vi "Populate 32-bit Block Memory.vi"(9 "Number of U32 words in Array":i32, 10 "Boolean array Block Mem in":refnum<k21>="Boolean Array", 11 "U32 Block Mem in":refnum<k21>) -> (3 "U32 Block mem Out":refnum<k21>)   [LabVIEW 2014]
uses:
  <vilib>/rvi/DataTransferAndStorage/Container/Common/niFpgaContainerExecOnDevCompGetState.vi
  <vilib>/rvi/Emulation/niFpgaEmulationIsFPGAContextNoSignature.vi
  <vilib>/rvi/DataTransferAndStorage/Container/Common/niFpgaContainerGetUniqueNameForEmu.vi
  <vilib>/rvi/Emulation/niFpgaProcessEmulError.vi
  <vilib>/rvi/Emulation/niFpgaSctlEmulationGetInTimedLoop.vi
  <vilib>/rvi/errors/nirviReportUnexpectedCaseInternalError (U32).vi
  <vilib>/rvi/Memory/Memory_Emulation/niFpgaMemoryEmulationCacheClearOnFirstRun.vi
  <vilib>/rvi/Memory/Memory_Emulation/nirvimemoryEmulationManagerCache_MakeExclusive.vi
  <vilib>/rvi/Memory/Memory_Emulation/niFpgaMemoryEmulationValidateCache.vi
  <vilib>/rvi/Memory/Memory_Emulation/nirvimemoryEmulationManagerCache_InsertValue.vi
  <vilib>/Utility/error.llb/Clear Errors.vi
  <vilib>/rvi/Memory/Memory_Emulation/nirvimemoryEmulationManagerCache_ReleaseExclusive.vi
  <vilib>/rvi/Memory/Memory_Emulation/nirvimemoryEmulationManagerCache_GetValue.vi
  <vilib>/rvi/Memory/Memory_Emulation/nirvimemoryEmulationManagerCache_SetValue.vi
  <vilib>/rvi/Emulation/niFpgaSctlEmulationResourceMgr.vi
  <vilib>/rvi/DataTransferAndStorage/Container/XNode/niFpgaContainer.xnode
  <vilib>/rvi/Memory/Memory_Emulation/niFpgaMemoryEmulationRefIn.vi
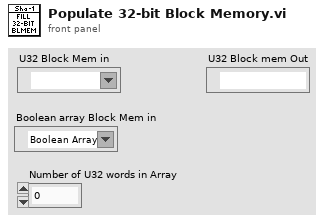
[diagram p1: front panel]
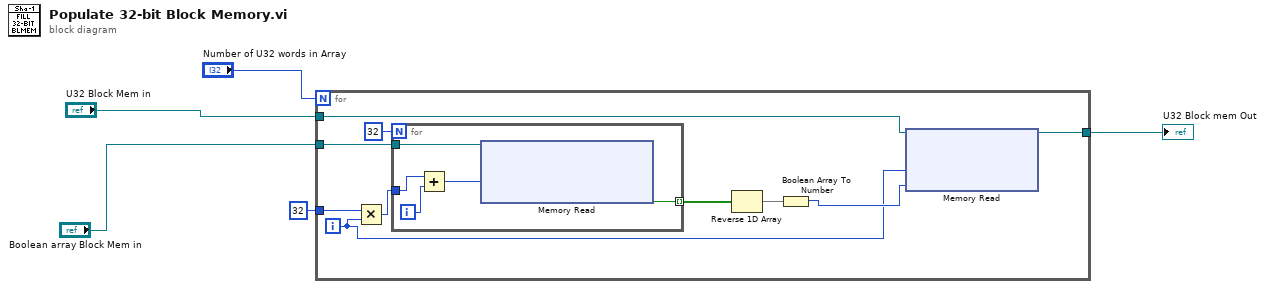
[diagram p0: block diagram]
diagram:
  n1 = for {
    N: "Number of U32 words in Array" -> [_]
    tunnel: "Boolean array Block Mem in" -> [w15]
    tunnel: 32 ("dimension size") -> [w11]
    tunnel: "U32 Block Mem in" -> [w9]
    tunnel: [w6] -> w5
    i -> [w7]
    n2 = Multiply(x=w11, y=w7) -> (x*y=w10:i32)
    n3 = for {
      N: 32 -> [_]
      tunnel: w15 -> [w20]
      tunnel: [w19] -> w13 mode=indexing
      tunnel: w10 -> [w17]
      i -> [w18]
      n4 = Add(x=w17, y=w18) -> (x+y=w16:i32)
      n5 = xnode ("Memory Read")("Address"=w16, "Memory In"=w20) -> ("Data"=w19:bool)  [unwired: 1 out]
    }
    n6 = Reverse 1D Array(array=w13) -> (reversed array=w12:bool[])
    n7 = Boolean Array To Number(Boolean array=w12) -> (number=w8:u32)
    n8 = xnode ("Memory Read")("Address"=w7, "Data"=w8, "Memory In"=w9) -> ("Memory Out"=w6:refnum<k21>)
  }
  "U32 Block mem Out" <- w5
